vi "sign_V.vi"(1 "输入":i8[](array[numeric])) -> (0 "输出":i8[](array[numeric]))   [LabVIEW 2018]
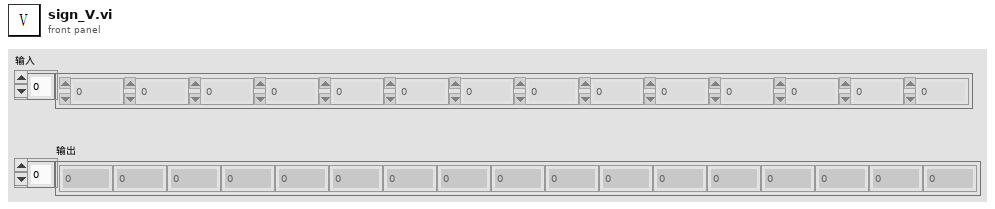
[diagram p1: front panel]
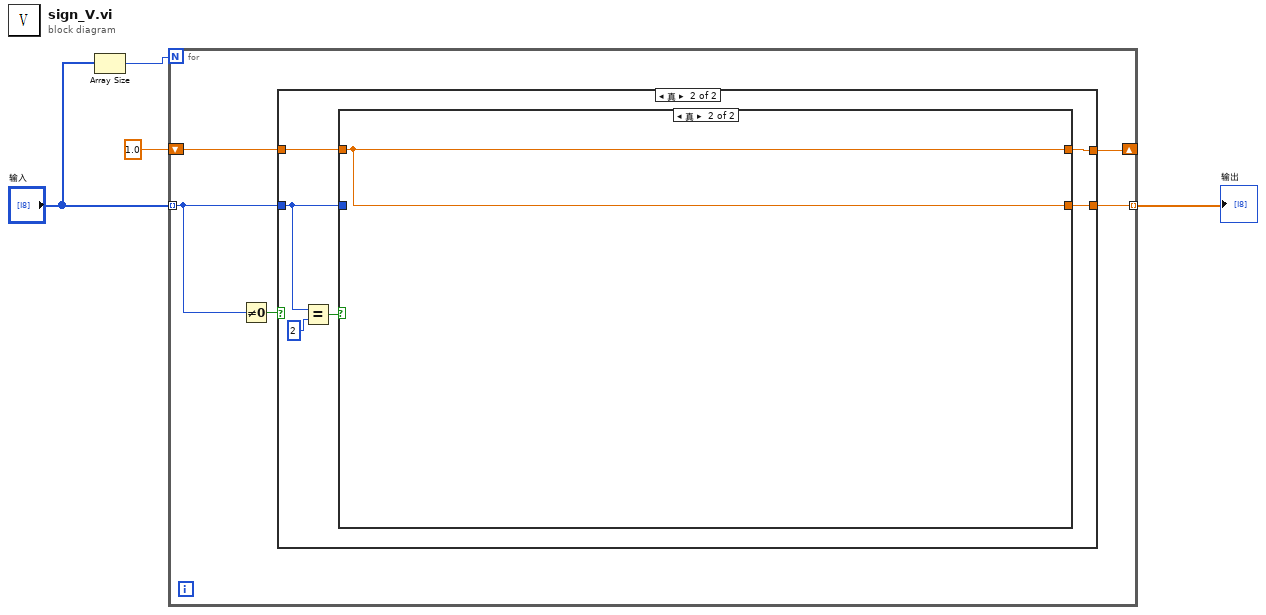
[diagram p0: block diagram]
diagram:
  n1 = Array Size(array="输入") -> (size(s)=w4:i32)
  n2 = for {
    N: w4 -> [_]
    tunnel: "输入" -> [w6] mode=indexing
    shift-right: [w7] -> _
    shift-left: 1.0 -> [w8]
    tunnel: [w5] -> w1 mode=indexing
    n3 = Not Equal To 0?(x=w6) -> (x != 0?=w9:bool)
    n4 = case shown="真" w9 {
      tunnel: [w11 w13] -> w7
      tunnel: w8 -> [w11 w15]
      tunnel: w6 -> [w10 w12]
      tunnel: [w10 w14] -> w5
      frame False {
      }
      frame True {
        n5 = Equal?(x=w12, y=i8 2) -> (x = y?=w17:bool)
        n6 = case shown="真" w17 {
          tunnel: w15 -> [_ w19]
          tunnel: [w18 w19] -> w14
          tunnel: [w18 w19] -> w13
          tunnel: w12 -> [w18 _]
          frame False {
          }
          frame True {
          }
        }
      }
    }
  }
  "输出" <- w1
